vi "SetRunOptions.vi"(7 "Options":T1={"exclude instances?"=FALSE, "exclude external? (T)"=TRUE, "separate tests?"=FALSE, "export dependencies?"=FALSE, "export rules?"=FALSE, "export invalid deps?"=FALSE, "export concessions?"=FALSE, "export undeclared?"=FALSE}, 8 "error in (no error)":errorcluster, 10 "Root path":path, 11 "CDependencyInspection in":refnum<class "CDependencyInspection.lvclass">) -> (0 "error out":errorcluster, 3 "CDependencyInspection out":refnum<class "CDependencyInspection.lvclass">)   [LabVIEW 2020, in "DependencyInspection.lvlib" / "CDependencyInspection.lvclass"]
uses:
  CDependencyInspection.lvclass
  Helper/subOptions.ctl
  CDependencyInspection.lvclass/CDependencyInspection.ctl
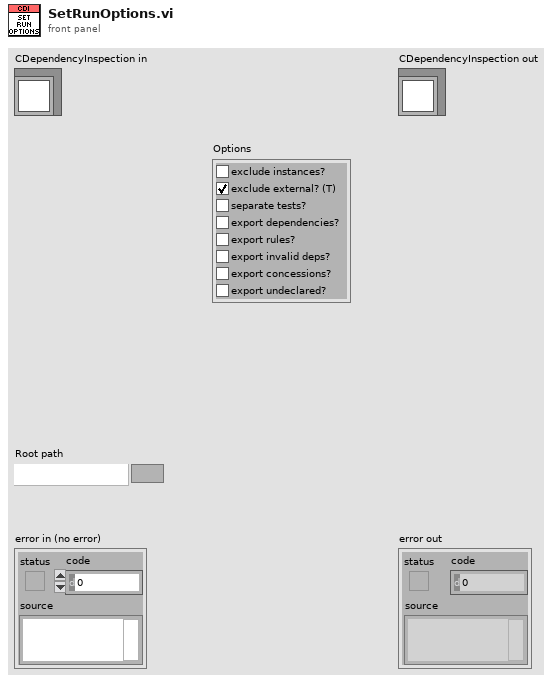
[diagram p1: front panel]
types:
  T1 = typedef "DependencyInspection.lvlib/CDependencyInspection.lvclass/subOptions.ctl" = cluster{"exclude instances?":bool, "exclude external? (T)":bool, "separate tests?":bool, "export dependencies?":bool, "export rules?":bool, "export invalid deps?":bool, "export concessions?":bool, "export undeclared?":bool}
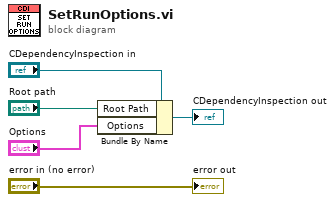
[diagram p0: block diagram]
diagram:
  n1 = Bundle By Name(cluster="CDependencyInspection in", "Root Path"="Root path", "Options"="Options") -> (→"CDependencyInspection out":refnum<class "CDependencyInspection.lvclass">)
  "error out" <- "error in (no error)"
